vi "Periodic Tasks.vi"(8 "error in":errorcluster) -> ()   [LabVIEW 2019]
doc: "This VI runs in parallel to other tasks. It can contain as many user-defined periodic loops as you need. These can carry out PID or other sorts of timed response."
uses:
  Classes/Logger/Type Defs/Logging Level.ctl
  TypeDefs/Falcon Temperatures.ctl
  RobotGlobal.vi
  <vilib>/Rock Robotics/Network Tables/NT Write Numeric Array.vi
  Classes/Drive/Tank Drive/Tank Drive.lvclass
  Classes/Logger/Logger.lvclass
  Classes/Turret/Turret.lvclass
  Classes/PowerCellHandler/Power Cell Handler.lvclass
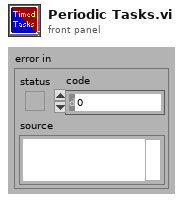
[diagram p1: front panel]
types:
  T1 = typedef "Falcon Temperatures.ctl" = enum16{"Accelerator", "Turret", "Flywheel", "Right follow", "Right lead", "Left follow", "Left lead"}
  T2 = typedef "Logger.lvlib/Logger.lvclass/Logging Level.ctl" = enum16{"Error", "Warning", "Info", "Trace"}
  T3 = typedef "RobotObjects.ctl" = cluster{"Drive.lvclass":refnum<class "Tank Drive.lvclass">, "Pneumatics.lvclass":refnum<class "Pneumatics.lvclass">, "Vision.lvclass":refnum<class "Vision.lvclass">, "Joysticks.lvclass":refnum<class "Joysticks.lvclass">, "Elevator.lvclass":refnum<class "Elevator.lvclass">, "Hatch.lvclass":refnum<class "Hatch.lvclass">, "Cargo.lvclass":refnum<class "Cargo.lvclass">, "DriveOld.lvclass":refnum<class "Drive.lvclass">, "Robot.lvclass":refnum<class "Robot.lvclass">, "Control Panel.lvclass":refnum<class "Control Panel.lvclass">, "Climber.lvclass":refnum<class "Climber.lvclass">, "Turret.lvlib:Turret.lvclass":refnum<class "Turret.lvclass">, "Power Cell Handler.lvclass":refnum<class "Power Cell Handler.lvclass">}
  T4 = typedef "Drive.lvlib/Tank Drive.lvclass/Drive Train Temperatures.ctl" = cluster{"Left Lead Temperature (C)":dbl, "Right Lead Temperature (C)":dbl, "Left Follows Temperatures (C)":dbl[], "Right Follows Temperatures (C)":dbl[]}
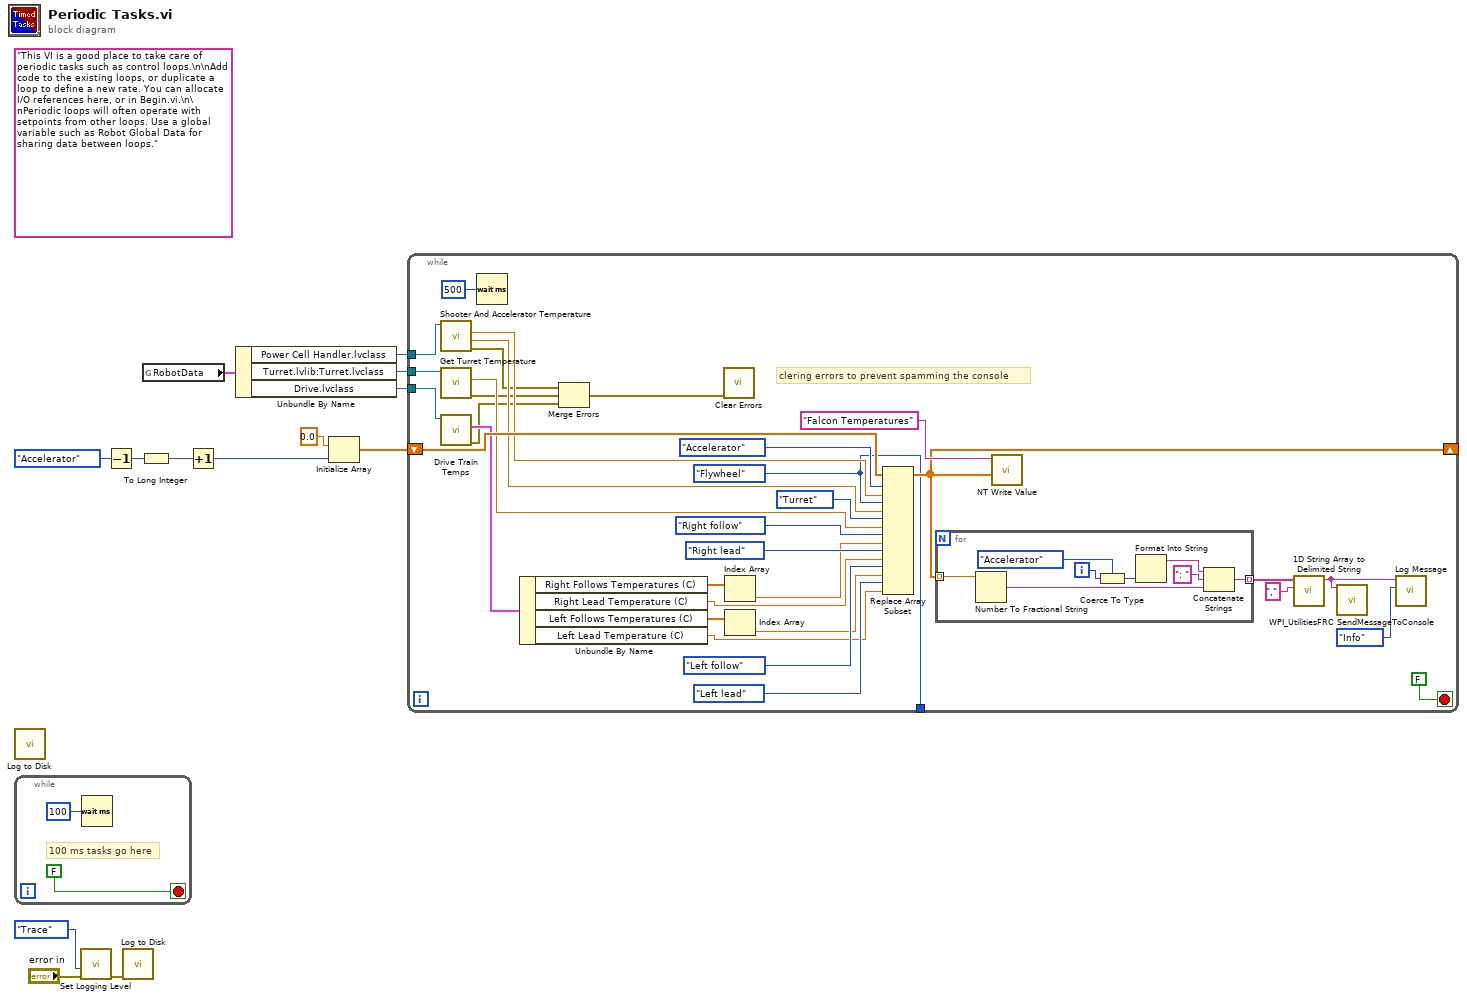
[diagram p0: block diagram]
diagram:
  (unwired) "This VI is a good place to take care of periodic tasks such as control loops.\n\nAdd code to the existing loops, or duplicate a loop to define a new rate. You can allocate I/O references here, or in Begin.vi.\n\nPeriodic loops will often operate with setpoints from other loops. Use a global variable such as Robot Global Data for sharing data between loops."
  n1 = call "Log to Disk.vi"() -> ()  [unwired: 12 in]
  n2 = while {
    stop <- FALSE stop-if-true
    # "100 ms tasks go here"
    n3 = Wait (ms)(milliseconds to wait=u32 100) -> ()  [unwired: 1 out]
  }
  n4 = call "Set Logging Level.vi"("error in (no error)"="error in", "Logging Level"=Logging_Level."Trace") -> ("error out"=w13:errorcluster)  [unwired: 9 in]
  n5 = Decrement(x=Falcon_Temperatures."Accelerator" ("Enum")) -> (x-1=w9:T1)
  n6 = call "Log to Disk.vi"("error in (no error)"=w13) -> ()  [unwired: 11 in]
  n7 = To Long Integer(number=w9) -> (32bit integer=w2:i32)
  n8 = global read "RobotGlobal.vi" "RobotData"() -> (w6:T3)
  n9 = Increment(x=w2) -> (x+1=w1:i32)
  n10 = Unbundle By Name(w6) -> ("Power Cell Handler.lvclass"=w3:refnum<class "Power Cell Handler.lvclass">, "Turret.lvlib:Turret.lvclass"=w5:refnum<class "Turret.lvclass">, "Drive.lvclass"=w4:refnum<class "Tank Drive.lvclass">)
  n11 = Initialize Array(0.0 ("element"), w1) -> (w7:dbl[])
  n12 = while {
    shift-right: [w22] -> _
    shift-left: w7 -> [w46]
    tunnel: w5 -> [w40]
    tunnel: w4 -> [w34]
    tunnel: w3 -> [w36]
    tunnel: [w16] -> _
    stop <- FALSE stop-if-true
    w16 = Falcon_Temperatures."Flywheel" ("Enum")
    # "clering errors to prevent spamming the console"
    n13 = call "Shooter And Accelerator Temperature.vi"("Power Cell Handler in"=w36) -> ("error out"=w25:errorcluster, "Shooter Temperature (C)"=w32:dbl, "Accelerator Temperature (C)"=w35:dbl)  [unwired: 7 in, 1 out]
    n14 = call "Get Turret Temperature.vi"("Turret in"=w40) -> ("error out"=w24:errorcluster, "Turret Temperature (C)"=w37:dbl)  [unwired: 8 in, 1 out]
    n15 = call-dynamic "Drive Train Temps.vi"("Tank Drive in"=w34) -> ("error out"=w23:errorcluster, "Drive Train Temperatures"=w33:T4)  [unwired: 8 in, 1 out]
    n16 = Wait (ms)(milliseconds to wait=u32 500) -> ()  [unwired: 1 out]
    n17 = Unbundle By Name(w33) -> ("Right Follows Temperatures (C)"=w31:dbl[], "Right Lead Temperature (C)"=w28:dbl, "Left Follows Temperatures (C)"=w30:dbl[], "Left Lead Temperature (C)"=w26:dbl)
    n18 = Merge Errors(w25, w24, w23) -> (w17:errorcluster)
    n19 = call <vilib>:"Clear Errors.vi"("error in (no error)"=w17) -> ()  [unwired: 5 in, 2 out]
    n20 = Index Array(array=w31) -> (element=w29:dbl)  [unwired: 1 in]
    n21 = Index Array(array=w30) -> (element=w27:dbl)  [unwired: 1 in]
    n22 = Replace Array Subset(array=w46, new element #1=w35, index #1=Falcon_Temperatures."Accelerator" ("Enum"), new element #2=w32, index #2=w16, new element #3=w37, index #3=Falcon_Temperatures."Turret" ("Enum"), new element #4=w29, index #4=Falcon_Temperatures."Right follow" ("Enum"), new element #5=w28, index #5=Falcon_Temperatures."Right lead" ("Enum"), new element #6=w27, index #6=Falcon_Temperatures."Left follow" ("Enum"), new element #7=w26, index #7=Falcon_Temperatures."Left lead" ("Enum")) -> (w22:dbl[])
    n23 = for {
      tunnel: w22 -> [w50] mode=indexing
      tunnel: [w49] -> w21 mode=indexing
      i -> [w54]
      n24 = Number To Fractional String(number=w50) -> (F-format string=w51:string)  [unwired: 3 in]
      n25 = Coerce To Type(0:w54, 1:Falcon_Temperatures."Accelerator" ("Enum")) -> (2:w56:T1)
      n26 = Format Into String(w56) -> (resulting string=w53:string)  [unwired: 3 in, 1 out]
      n27 = Concatenate Strings(w53, ": " ("string"), w51) -> (w49:string)
    }
    n28 = call-poly <vilib>:"NT Write Value.vi"("Numeric Array"=w22, "Name"="Falcon Temperatures") -> ()  [unwired: 9 in, 1 out]
    n29 = call <vilib>:"1D String Array to Delimited String.vi"("delimiter"="," ("delimiter (\\t)"), "string array"=w21) -> ("delimited string"=w18:string)  [unwired: 9 in]
    n30 = call <vilib>:"WPI_UtilitiesFRC SendMessageToConsole.vi"("Message"=w18) -> ()  [unwired: 14 in, 1 out]
    n31 = call "Log Message.vi"("Logging Level"=Logging_Level."Info", "Message"=w18) -> ()  [unwired: 9 in, 1 out]
  }
